vi "Variant to LVOBJ.vi"(8 "error in (no error)":errorcluster, 10 "Enums as string? (F)":bool, 11 "Variant in":variant) -> (0 "error out":errorcluster, 3 "Root":T1)   [LabVIEW 2019, in "labview_json.lvlib"]
uses:
  labview_json.lvlib
  Value.ctl
  Value Type.ctl
  <vilib>/Utility/error.llb/Error Cluster From Error Code.vi
  <vilib>/ErrorRing/Error Ring.xnode
  <vilib>/Utility/Data Type/NI_Data Type.lvlib
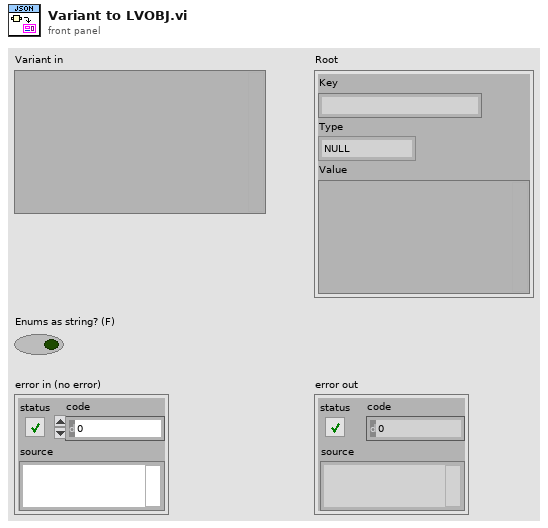
[diagram p1: front panel]
types:
  T1 = typedef "labview_json.lvlib/Value.ctl" = cluster{"Key":string, "Type":T2, "Value":variant}
  T2 = typedef "labview_json.lvlib/Value Type.ctl" = enum8{"NULL", "OBJECT", "ARRAY", "BOOL", "INT", "UINT", "FLOAT", "STRING"}
  T3 = typedef "NI_Data Type.lvlib/Data Type.ctl" = enum8{"Invalid Type", "Void", "I8", "I16", "I32", "I64", "U8", "U16", "U32", "U64", "Single Float", "Double Float", "Extended Float", "Single Complex", "Double Complex", "Extended Complex", "Enum U8", "Enum U16", "Enum U32", "Enum U64", "Single Float With Unit", "Double Float With Unit", "Extended Float With Unit", "Single Complex with Unit", "Double Complex with Unit", "Extended Complex with Unit", "Boolean", "String", "Path", "Picture", "Tag", "Array", "Cluster", "Variant", "LV Variant", "Waveform", "Timestamp", "Digital Waveform", "Digital Data", "ExpressData", "Refnum", "External Data", "VI", "Poly VI", "LabVIEW Class Instance", "Fixed Point", "Set Collection", "Map Collection"}
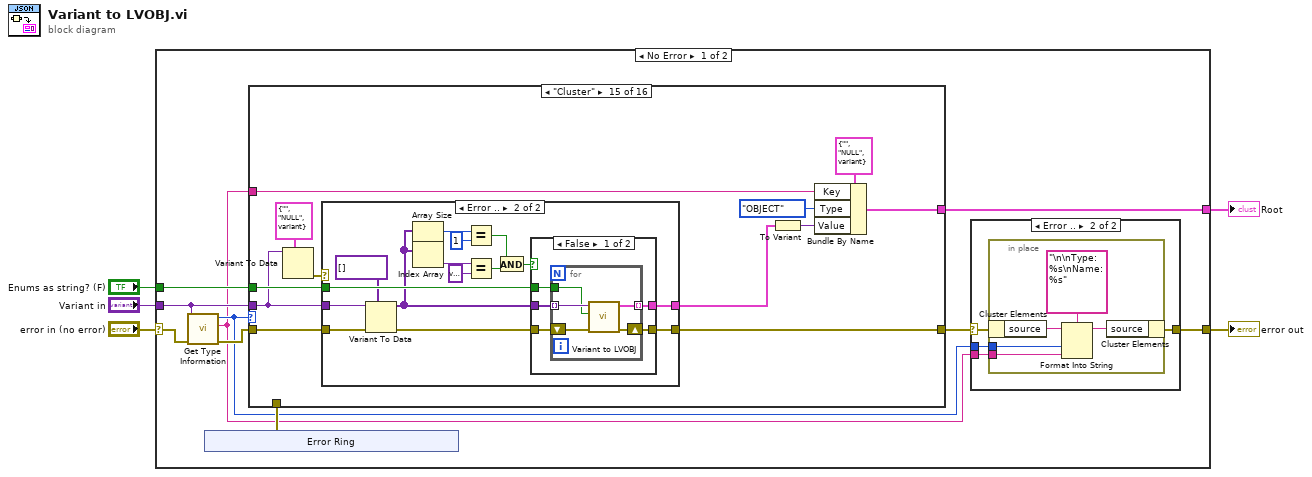
[diagram p0: block diagram]
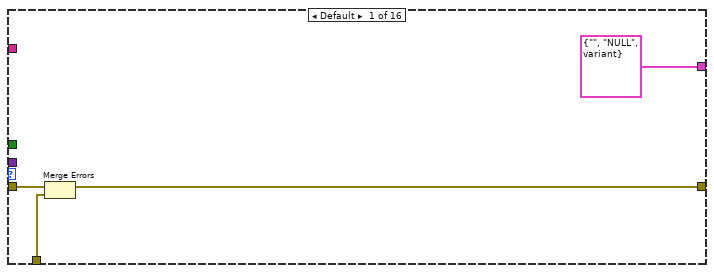
[diagram p2: hidden frame]
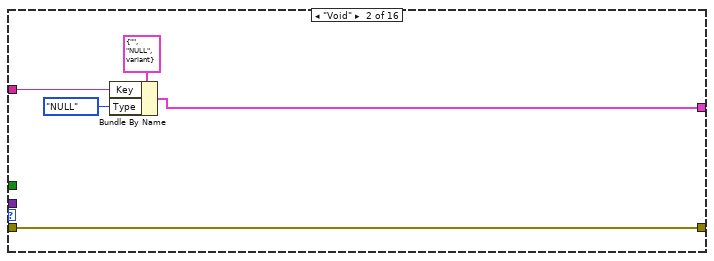
[diagram p3: hidden frame]
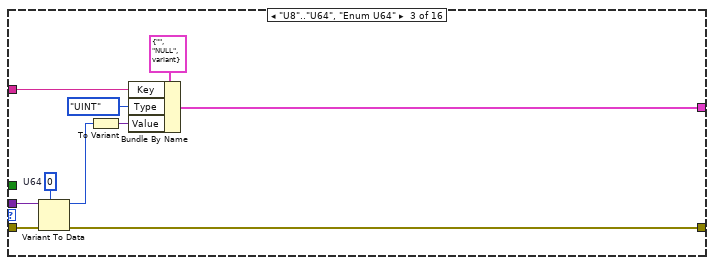
[diagram p4: hidden frame]
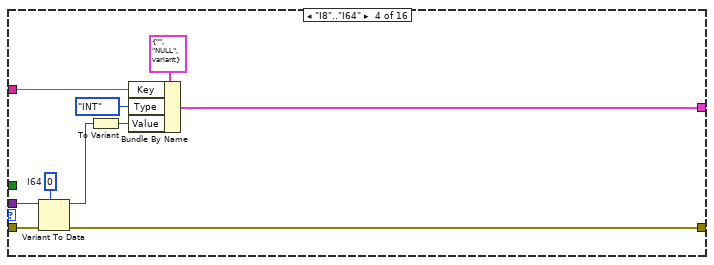
[diagram p5: hidden frame]
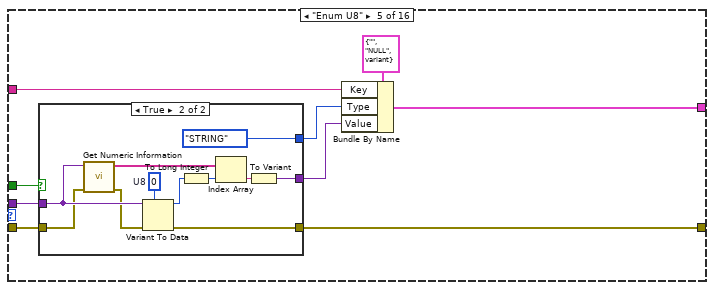
[diagram p6: hidden frame]
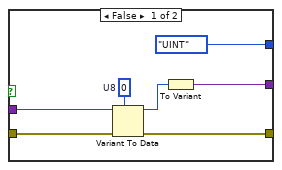
[diagram p7: hidden frame]
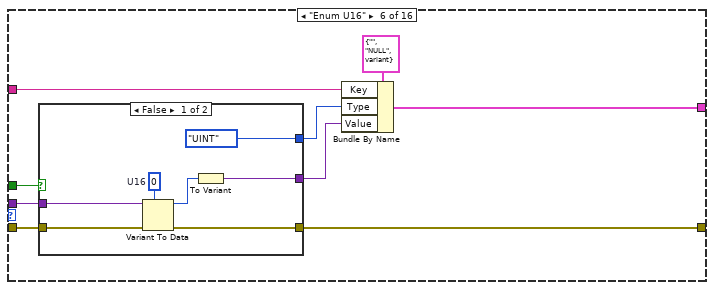
[diagram p8: hidden frame]
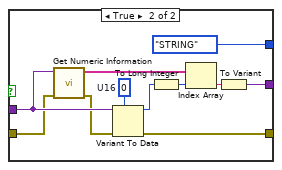
[diagram p9: hidden frame]
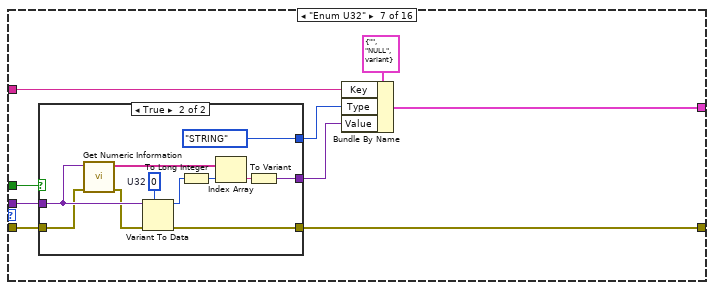
[diagram p10: hidden frame]
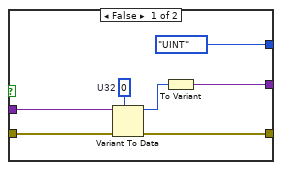
[diagram p11: hidden frame]
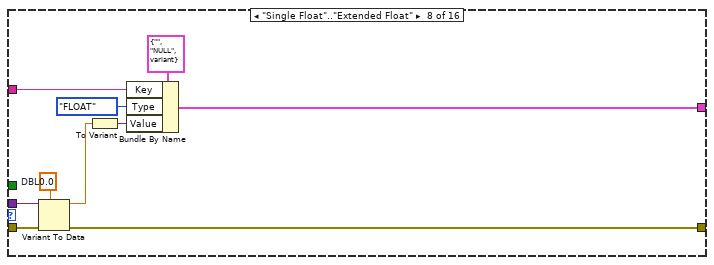
[diagram p12: hidden frame]
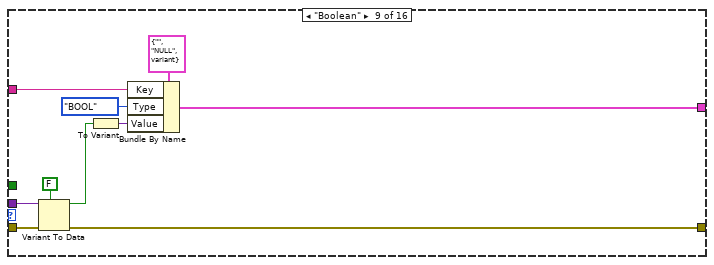
[diagram p13: hidden frame]
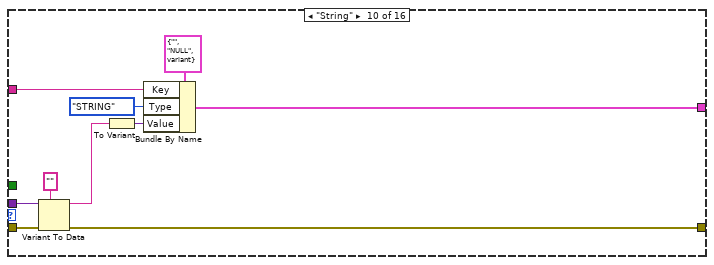
[diagram p14: hidden frame]
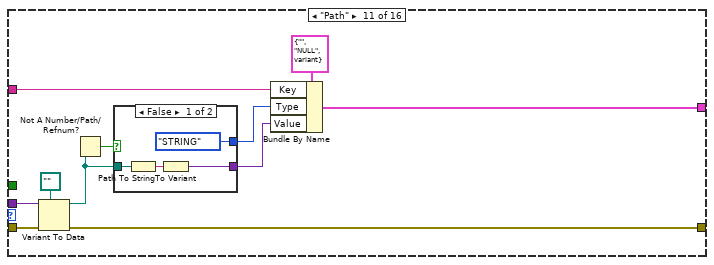
[diagram p15: hidden frame]
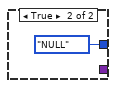
[diagram p16: hidden frame]
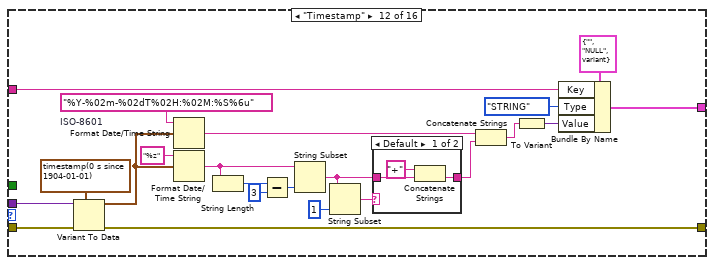
[diagram p17: hidden frame]
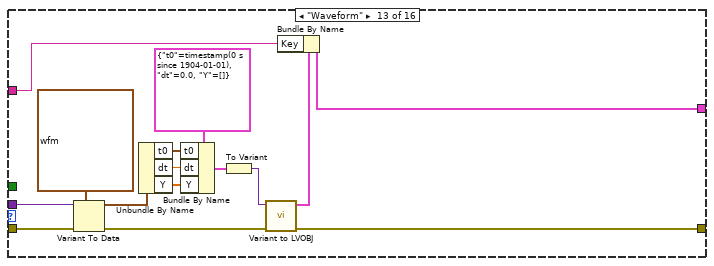
[diagram p19: hidden frame]
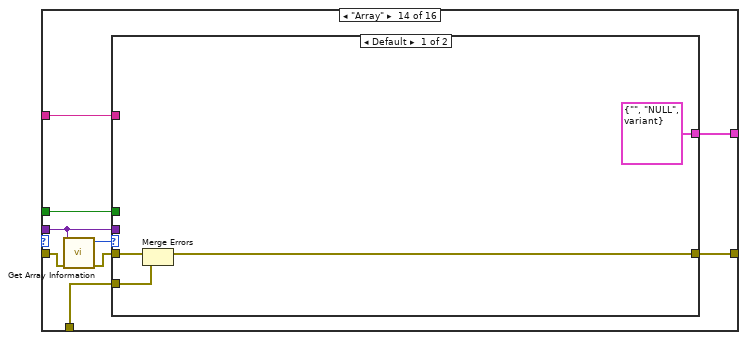
[diagram p20: hidden frame]
diagram:
  n1 = case shown="No Error" "error in (no error)" {
    selector: "error in (no error)" -> [w15 w311]
    tunnel: "Variant in" -> [w13 _]
    tunnel: [w8 w311] -> w3
    tunnel: [w12 T1 {"Key"="", "Type"=enum."NULL", "Value"=variant} ("Root")] -> w1
    tunnel: "Enums as string? (F)" -> [w10 _]
    frame No Error {
      n2 = call <vilib>:"Get Type Information.vi"("error in (no error)"=w15, "variant"=w13) -> ("error out"=w14:errorcluster, "name"=w6:string, "type"=w7:T3)  [unwired: 5 in, 2 out]
      n3 = xnode "Error Ring"() -> ("error out"=w11:errorcluster)
      n4 = case shown="\"Cluster\"" w7 {
        tunnel: w14 -> [w19 w24 w34 w44 w53 w80 w107 w135 w145 w155 w166 w193 w212 w221 w253 w288]
        tunnel: w13 -> [_ _ w33 w43 w52 w79 w106 w134 w144 w154 w165 w192 w211 w216 w246 w287]
        tunnel: [w17 w24 w31 w41 w51 w78 w105 w132 w143 w153 w164 w191 w203 w218 w255 w288] -> w9
        tunnel: [T1 {"Key"="", "Type"=enum."NULL", "Value"=variant} ("Root") w22 w29 w39 w48 w75 w102 w126 w136 w146 w157 w172 w199 w214 w247 w289] -> w12
        tunnel: w11 -> [w18 _ _ _ _ _ _ _ _ _ _ _ _ w217 _ _]
        tunnel: w10 -> [_ _ _ _ w50 w77 w104 _ _ _ _ _ _ w215 w254 _]
        tunnel: w6 -> [_ w21 w28 w38 w46 w73 w100 w130 w138 w148 w159 w175 w198 w213 w249 w290]
        frame Default {
          n5 = Merge Errors(w19, w18) -> (w17:errorcluster)
        }
        frame "Void" {
          n6 = Bundle By Name(cluster=T1 {"Key"="", "Type"=enum."NULL", "Value"=variant} ("Root"), "Key"=w21, "Type"=Value_Type."NULL") -> (w22:T1)
        }
        frame "U8".."U64", "Enum U64" {
          w32 = u64 0  # U64
          n7 = Variant To Data(error in=w34, type=w32, Variant=w33) -> (data=w26:u64, error out=w31:errorcluster)
          n8 = To Variant(anything=w26) -> (Variant=w25:variant)
          n9 = Bundle By Name(cluster=T1 {"Key"="", "Type"=enum."NULL", "Value"=variant} ("Root"), "Key"=w28, "Type"=Value_Type."UINT", "Value"=w25) -> (w29:T1)
        }
        frame "I8".."I64" {
          w42 = i64 0  # I64
          n10 = Variant To Data(error in=w44, type=w42, Variant=w43) -> (data=w36:i64, error out=w41:errorcluster)
          n11 = To Variant(anything=w36) -> (Variant=w35:variant)
          n12 = Bundle By Name(cluster=T1 {"Key"="", "Type"=enum."NULL", "Value"=variant} ("Root"), "Key"=w38, "Type"=Value_Type."INT", "Value"=w35) -> (w39:T1)
        }
        frame "Enum U8" {
          n13 = case shown="True" w50 {
            tunnel: w53 -> [w60 w65]
            tunnel: w52 -> [w59 w69]
            tunnel: [w57 w70] -> w51
            tunnel: [w55 w62] -> w47
            tunnel: [Value_Type."UINT" ("Type") Value_Type."STRING" ("Type")] -> w45
            frame False {
              w58 = u8 0  # U8
              n14 = Variant To Data(error in=w60, type=w58, Variant=w59) -> (data=w56:u8, error out=w57:errorcluster)
              n15 = To Variant(anything=w56) -> (Variant=w55:variant)
            }
            frame True {
              w71 = u8 0  # U8
              n16 = call <vilib>:"Get Numeric Information.vi"("error in (no error)"=w65, "variant"=w69) -> ("error out"=w66:errorcluster, "enum names"=w68:string[])  [unwired: 6 in, 2 out]
              n17 = Variant To Data(error in=w66, type=w71, Variant=w69) -> (data=w67:u8, error out=w70:errorcluster)
              n18 = To Long Integer(number=w67) -> (32bit integer=w64:i32)
              n19 = Index Array(array=w68, index=w64) -> (element=w63:string)
              n20 = To Variant(anything=w63) -> (Variant=w62:variant)
            }
          }
          n21 = Bundle By Name(cluster=T1 {"Key"="", "Type"=enum."NULL", "Value"=variant} ("Root"), "Key"=w46, "Type"=w45, "Value"=w47) -> (w48:T1)
        }
        frame "Enum U16" {
          n22 = case shown="False" w77 {
            tunnel: w80 -> [w87 w92]
            tunnel: w79 -> [w86 w96]
            tunnel: [w84 w97] -> w78
            tunnel: [w82 w89] -> w74
            tunnel: [Value_Type."UINT" ("Type") Value_Type."STRING" ("Type")] -> w72
            frame False {
              w85 = u16 0  # U16
              n23 = Variant To Data(error in=w87, type=w85, Variant=w86) -> (data=w83:u16, error out=w84:errorcluster)
              n24 = To Variant(anything=w83) -> (Variant=w82:variant)
            }
            frame True {
              w98 = u16 0  # U16
              n25 = call <vilib>:"Get Numeric Information.vi"("error in (no error)"=w92, "variant"=w96) -> ("error out"=w93:errorcluster, "enum names"=w95:string[])  [unwired: 6 in, 2 out]
              n26 = Variant To Data(error in=w93, type=w98, Variant=w96) -> (data=w94:u16, error out=w97:errorcluster)
              n27 = To Long Integer(number=w94) -> (32bit integer=w91:i32)
              n28 = Index Array(array=w95, index=w91) -> (element=w90:string)
              n29 = To Variant(anything=w90) -> (Variant=w89:variant)
            }
          }
          n30 = Bundle By Name(cluster=T1 {"Key"="", "Type"=enum."NULL", "Value"=variant} ("Root"), "Key"=w73, "Type"=w72, "Value"=w74) -> (w75:T1)
        }
        frame "Enum U32" {
          n31 = case shown="True" w104 {
            tunnel: w107 -> [w114 w119]
            tunnel: w106 -> [w113 w123]
            tunnel: [w111 w124] -> w105
            tunnel: [w109 w116] -> w101
            tunnel: [Value_Type."UINT" ("Type") Value_Type."STRING" ("Type")] -> w99
            frame False {
              w112 = u32 0  # U32
              n32 = Variant To Data(error in=w114, type=w112, Variant=w113) -> (data=w110:u32, error out=w111:errorcluster)
              n33 = To Variant(anything=w110) -> (Variant=w109:variant)
            }
            frame True {
              w125 = u32 0  # U32
              n34 = call <vilib>:"Get Numeric Information.vi"("error in (no error)"=w119, "variant"=w123) -> ("error out"=w120:errorcluster, "enum names"=w122:string[])  [unwired: 6 in, 2 out]
              n35 = Variant To Data(error in=w120, type=w125, Variant=w123) -> (data=w121:u32, error out=w124:errorcluster)
              n36 = To Long Integer(number=w121) -> (32bit integer=w118:i32)
              n37 = Index Array(array=w122, index=w118) -> (element=w117:string)
              n38 = To Variant(anything=w117) -> (Variant=w116:variant)
            }
          }
          n39 = Bundle By Name(cluster=T1 {"Key"="", "Type"=enum."NULL", "Value"=variant} ("Root"), "Key"=w100, "Type"=w99, "Value"=w101) -> (w102:T1)
        }
        frame "Single Float".."Extended Float" {
          w133 = 0.0  # DBL
          n40 = Variant To Data(error in=w135, type=w133, Variant=w134) -> (data=w129:dbl, error out=w132:errorcluster)
          n41 = To Variant(anything=w129) -> (Variant=w128:variant)
          n42 = Bundle By Name(cluster=T1 {"Key"="", "Type"=enum."NULL", "Value"=variant} ("Root"), "Key"=w130, "Type"=Value_Type."FLOAT", "Value"=w128) -> (w126:T1)
        }
        frame "Boolean" {
          n43 = Variant To Data(error in=w145, type=FALSE, Variant=w144) -> (data=w137:bool, error out=w143:errorcluster)
          n44 = To Variant(anything=w137) -> (Variant=w140:variant)
          n45 = Bundle By Name(cluster=T1 {"Key"="", "Type"=enum."NULL", "Value"=variant} ("Root"), "Key"=w138, "Type"=Value_Type."BOOL", "Value"=w140) -> (w136:T1)
        }
        frame "String" {
          n46 = Variant To Data(error in=w155, type="", Variant=w154) -> (data=w147:string, error out=w153:errorcluster)
          n47 = To Variant(anything=w147) -> (Variant=w150:variant)
          n48 = Bundle By Name(cluster=T1 {"Key"="", "Type"=enum."NULL", "Value"=variant} ("Root"), "Key"=w148, "Type"=Value_Type."STRING", "Value"=w150) -> (w146:T1)
        }
        frame "Path" {
          n49 = Variant To Data(error in=w166, type=path "", Variant=w165) -> (data=w162:path, error out=w164:errorcluster)
          n50 = Not A Number/Path/Refnum?(number/path/refnum=w162) -> (NaN/Path/Refnum?=w161:bool)
          n51 = case shown="False" w161 {
            tunnel: [w168 _] -> w158
            tunnel: w162 -> [w170 _]
            tunnel: [Value_Type."STRING" ("Type") Value_Type."NULL" ("Type")] -> w156
            frame False {
              n52 = Path To String(path=w170) -> (string=w169:string)
              n53 = To Variant(anything=w169) -> (Variant=w168:variant)
            }
            frame True {
            }
          }
          n54 = Bundle By Name(cluster=T1 {"Key"="", "Type"=enum."NULL", "Value"=variant} ("Root"), "Key"=w159, "Type"=w156, "Value"=w158) -> (w157:T1)
        }
        frame "Timestamp" {
          w189 = "%Y-%02m-%02dT%02H:%02M:%S%6u"  # ISO-8601
          n55 = Variant To Data(error in=w193, type=timestamp(0 s since 1904-01-01), Variant=w192) -> (data=w178:timestamp, error out=w191:errorcluster)
          n56 = Format Date/Time String(time format string (%c)=w189, seconds (now)=w178) -> (date/time string=w188:string)  [unwired: 1 in]
          n57 = Format Date/Time String(time format string (%c)="%z", seconds (now)=w178) -> (date/time string=w186:string)  [unwired: 1 in]
          n58 = String Length(string=w186) -> (length=w185:i32)
          n59 = Subtract(x=w185, y=3) -> (x-y=w183:i32)
          n60 = String Subset(string=w186, length (rest)=w183) -> (substring=w180:string)  [unwired: 1 in]
          n61 = String Subset(string=w180, length (rest)=1 ("length (rest)")) -> (substring=w181:string)  [unwired: 1 in]
          n62 = case shown="Default" w181 {
            tunnel: [w195 w197] -> w179
            tunnel: w180 -> [w196 w197]
            frame Default {
              n63 = Concatenate Strings("+" ("string"), w196) -> (w195:string)
            }
            frame "-" {
            }
          }
          n64 = Concatenate Strings(w188, w179) -> (w174:string)
          n65 = To Variant(anything=w174) -> (Variant=w173:variant)
          n66 = Bundle By Name(cluster=T1 {"Key"="", "Type"=enum."NULL", "Value"=variant} ("Root"), "Key"=w175, "Type"=Value_Type."STRING", "Value"=w173) -> (w172:T1)
        }
        frame "Waveform" {
          n67 = Variant To Data(error in=w212, type=waveform(dbl) {"t0"=timestamp(0 s since 1904-01-01), "dt"=1.0, "Y"=[]} ("Waveform"), Variant=w211) -> (data=w208:waveform(dbl), error out=w204:errorcluster)
          n68 = Unbundle By Name(w208) -> ("t0"=w207:timestamp, "dt"=w206:dbl, "Y"=w205:dbl[])
          n69 = Bundle By Name(cluster=cluster{"t0":timestamp, "dt":dbl, "Y":dbl[]} {"t0"=timestamp(0 s since 1904-01-01), "dt"=0.0, "Y"=[]} ("Waveform"), "t0"=w207, "dt"=w206, "Y"=w205) -> (w202:cluster{"t0":timestamp, "dt":dbl, "Y":dbl[]})
          n70 = To Variant(anything=w202) -> (Variant=w201:variant)
          n71 = call "Variant to LVOBJ.vi"("error in (no error)"=w204, "Variant in"=w201) -> ("error out"=w203:errorcluster, "Root"=w200:T1)  [unwired: 8 in]
          n72 = Bundle By Name(cluster=w200, "Key"=w198) -> (w199:T1)
        }
        frame "Array" {
          n73 = call <vilib>:"Get Array Information.vi"("error in (no error)"=w221, "variant"=w216) -> ("error out"=w219:errorcluster, "number of dimensions"=w220:i32)  [unwired: 6 in, 2 out]
          n74 = case shown="Default" w220 {
            tunnel: w219 -> [w225 w238]
            tunnel: [w224 w232] -> w218
            tunnel: w217 -> [w223 _]
            tunnel: w216 -> [_ w237]
            tunnel: w215 -> [_ w233]
            tunnel: [T1 {"Key"="", "Type"=enum."NULL", "Value"=variant} ("Root") w228] -> w214
            tunnel: w213 -> [_ w226]
            frame Default {
              n75 = Merge Errors(w225, w223) -> (w224:errorcluster)
            }
            frame 1 {
              n76 = Variant To Data(error in=w238, type=variant[] [], Variant=w237) -> (data=w234:variant[], error out=w235:errorcluster)
              n77 = for {
                tunnel: w234 -> [w242] mode=indexing
                tunnel: w233 -> [w241]
                shift-right: [w240] -> w232
                shift-left: w235 -> [w243]
                tunnel: [w239] -> w229 mode=indexing
                n78 = call "Variant to LVOBJ.vi"("error in (no error)"=w243, "Enums as string? (F)"=w241, "Variant in"=w242) -> ("error out"=w240:errorcluster, "Root"=w239:T1)  [unwired: 7 in]
              }
              n79 = To Variant(anything=w229) -> (Variant=w230:variant)
              n80 = Bundle By Name(cluster=T1 {"Key"="", "Type"=enum."NULL", "Value"=variant} ("Root"), "Key"=w226, "Type"=Value_Type."ARRAY", "Value"=w230) -> (w228:T1)
            }
          }
        }
        frame "Cluster" {
          n81 = Variant To Data(type=T1 {"Key"="", "Type"=enum."NULL", "Value"=variant} ("Root"), Variant=w246) -> (error out=w244:errorcluster)  [unwired: 1 in, 1 out]
          n82 = case shown="Error .." w244 {
            tunnel: [w256 w271] -> w255
            tunnel: w254 -> [_ w270]
            tunnel: w253 -> [w256 w267]
            tunnel: [_ w266] -> w248
            tunnel: w246 -> [_ w257]
            frame No Error {
            }
            frame Error {
              n83 = Variant To Data(error in=w267, type=variant[] [], Variant=w257) -> (data=w263:variant[], error out=w268:errorcluster)
              n84 = Array Size(array=w263) -> (size(s)=w265:i32)
              n85 = Index Array(array=w263) -> (element=w262:variant)  [unwired: 1 in]
              n86 = Equal?(x=w265, y=1) -> (x = y?=w259:bool)
              n87 = Equal?(x=w262, y=variant ("x")) -> (x = y?=w260:bool)
              n88 = And(x=w259, y=w260) -> (x .and. y?=w258:bool)
              n89 = case shown="False" w258 {
                tunnel: [w276 w282] -> w271
                tunnel: w270 -> [w275 _]
                tunnel: w268 -> [w274 w282]
                tunnel: [w273 _] -> w266
                tunnel: w263 -> [w272 _]
                frame False {
                  n90 = for {
                    tunnel: w272 -> [w280] mode=indexing
                    tunnel: w275 -> [w279]
                    shift-right: [w278] -> w276
                    shift-left: w274 -> [w281]
                    tunnel: [w277] -> w273 mode=indexing
                    n91 = call "Variant to LVOBJ.vi"("error in (no error)"=w281, "Enums as string? (F)"=w279, "Variant in"=w280) -> ("error out"=w278:errorcluster, "Root"=w277:T1)  [unwired: 7 in]
                  }
                }
                frame True {
                }
              }
            }
          }
          n92 = To Variant(anything=w248) -> (Variant=w251:variant)
          n93 = Bundle By Name(cluster=T1 {"Key"="", "Type"=enum."NULL", "Value"=variant} ("Root"), "Key"=w249, "Type"=Value_Type."OBJECT", "Value"=w251) -> (w247:T1)
        }
        frame "LV Variant" {
          n94 = Equal?(x=variant, y=w287) -> (x = y?=w285:bool)
          n95 = case shown="False" w285 {
            tunnel: [Value_Type."OBJECT" ("Type") Value_Type."NULL" ("Type")] -> w284
            tunnel: [w292 _] -> w283
            frame True {
              n96 = To Variant(anything=T1[] []) -> (Variant=w292:variant)
            }
            frame False {
            }
          }
          n97 = Bundle By Name(cluster=T1 {"Key"="", "Type"=enum."NULL", "Value"=variant} ("Root"), "Key"=w290, "Type"=w284, "Value"=w283) -> (w289:T1)
        }
      }
      n98 = case shown="Error .." w9 {
        selector: w9 -> [w296 w300]
        tunnel: [w296 w299] -> w8
        tunnel: w7 -> [_ w298]
        tunnel: w6 -> [_ w297]
        frame No Error {
        }
        frame Error {
          n99 = in-place {
            in-place-border: w298 -> [w302]
            in-place-border: w297 -> [w301]
            n100 = in-place-cluster #1(w300) -> ("source"=w305:string)
            n101 = Format Into String(format string="\n\nType: %s\nName: %s", initial string=w305, w302, w301) -> (resulting string=w304:string)  [unwired: 1 in, 1 out]
            n102 = in-place-cluster #1("source"=w304) -> (w299:errorcluster)
          }
        }
      }
    }
    frame Error {
    }
  }
  "error out" <- w3
  "Root" <- w1
